vi "New_GraphDispWithTime.vi"() -> ()   [LabVIEW 2016, in "PanelSplitForDisplay.lvclass"]
uses:
  PanelSplit/PanelSplitForDisplay.lvclass
  PanelSplit/PanelObject/PanelObject.lvclass
  <vilib>/Utility/error.llb/DialogType.ctl
  PanelSplit/PanelDataNode/PanelDataNode.lvclass
  Architecture/Queue Management/ARC_Queue Create_Single.vi
  Architecture/Queue Management/ARC_Queue Remove Element.vi
  Ctrls/GlobeVaribles.vi
  Architecture/Queue Management/ARC_Queue Insert Element.vi
  Architecture/Queue Management/ARC_Queue Destroy_Single.vi
panel:
  out "Y Scale.Scale Fit":u8
  out "size(s)":i32
  in  "Node*":refnum<data-value>
  out "Waveform Chart":waveform(dbl)(graph)
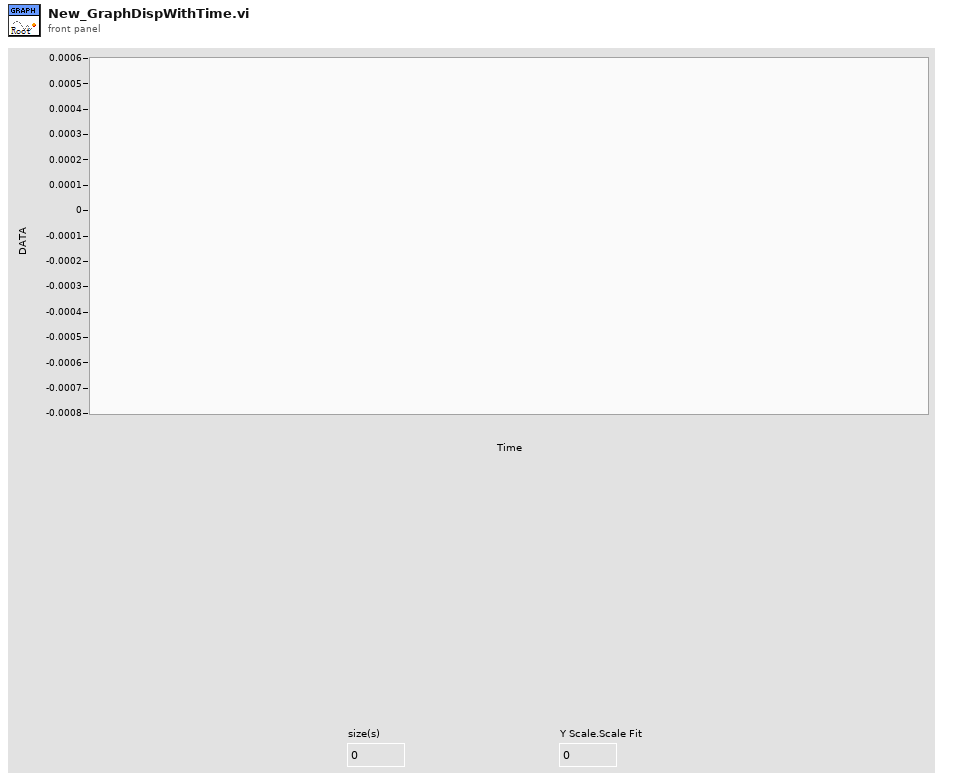
[diagram p1: front panel]
types:
  T1 = cluster{"error":errorcluster, "Event":string, "Data":variant, "Q_Local":string, "Graph":refnum<vi>, "Q_Caller":string}
  T2 = typedef "DialogType.ctl" = u16
  T3 = typedef "LVRectTypeDef.ctl" = cluster{"Left":i16, "Top":i16, "Right":i16, "Bottom":i16}
  T4 = typedef "PanelSplitForDisplay.lvclass/ViValueCtl.ctl" = cluster{"CHTag":string, "GraphProperts":cluster{"YMax":dbl, "YMin":dbl, "ScaleFit":u8}, "CHUnit":string, "CHName":string, "CHValue":string, "CHAlias":string}
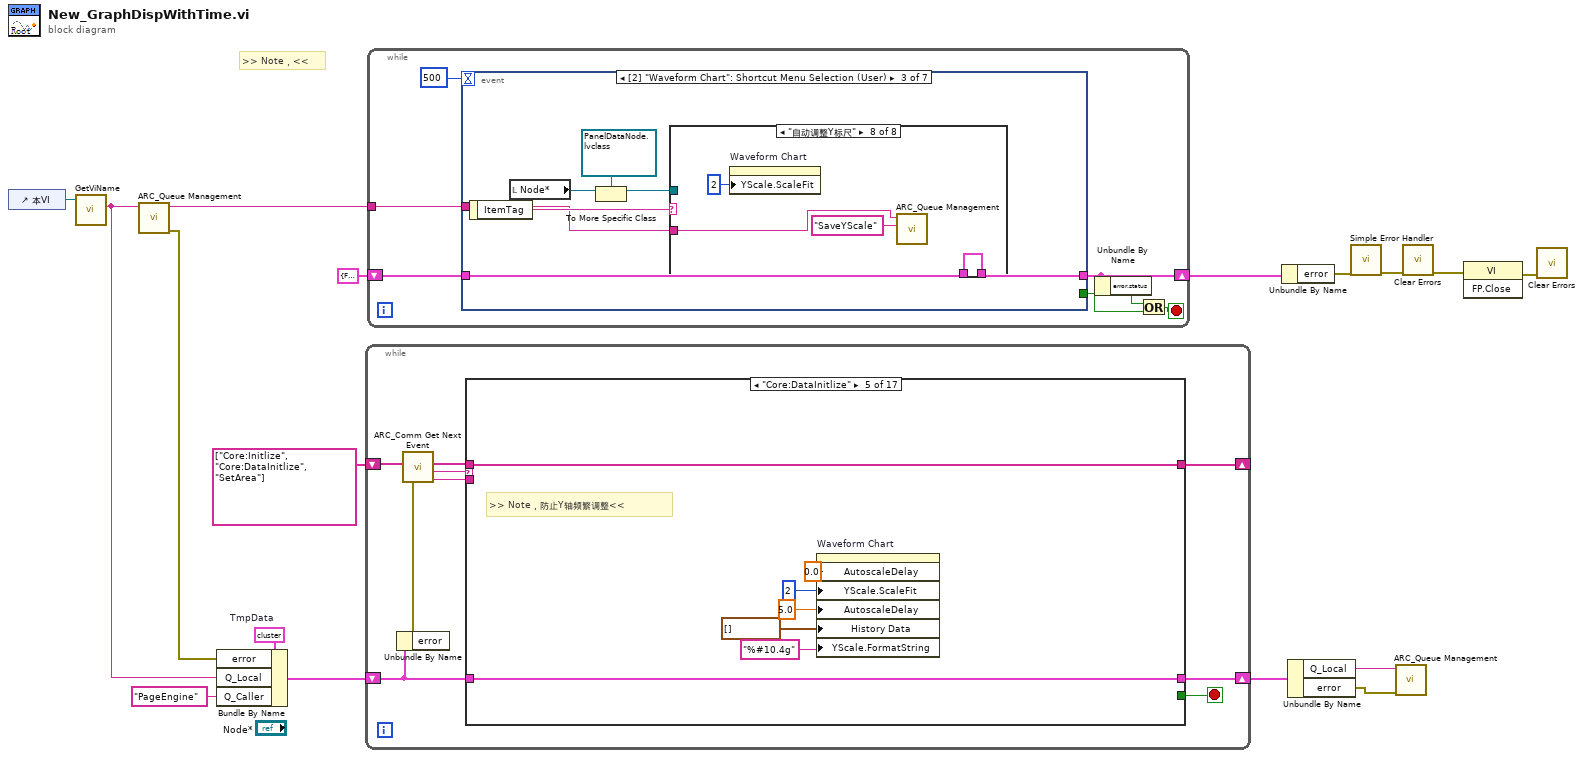
[diagram p0: block diagram]
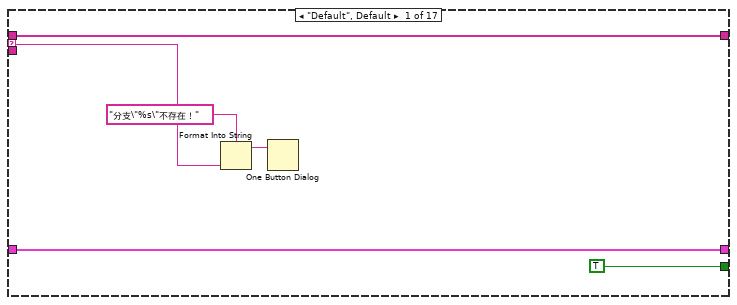
[diagram p2: hidden frame]
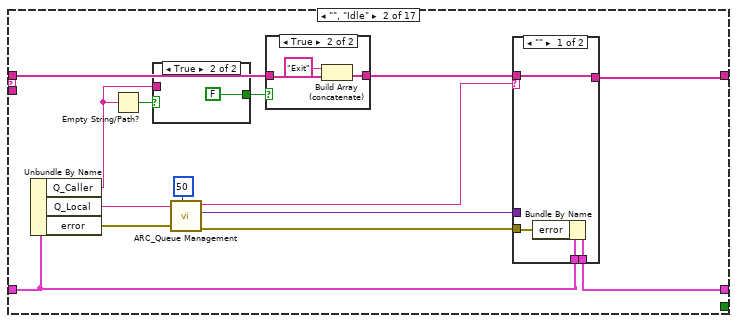
[diagram p3: hidden frame]
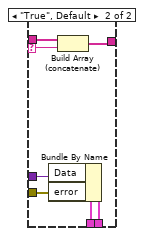
[diagram p4: hidden frame]
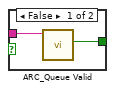
[diagram p6: hidden frame]
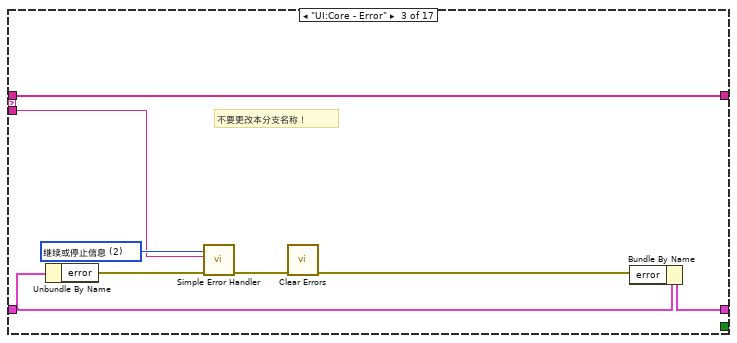
[diagram p7: hidden frame]
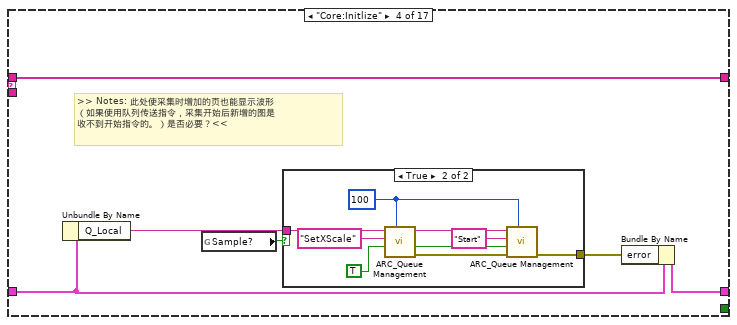
[diagram p8: hidden frame]
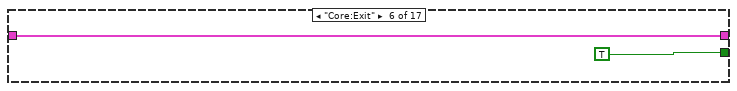
[diagram p10: hidden frame]
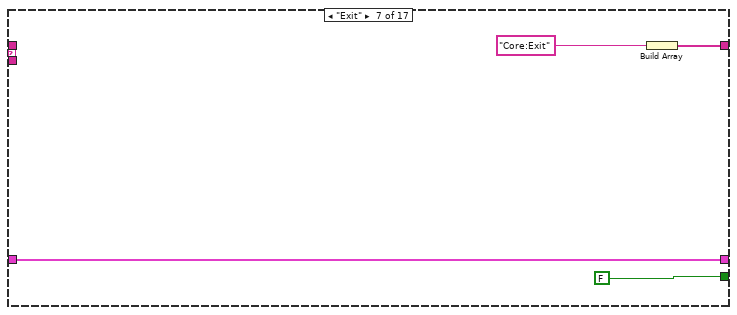
[diagram p11: hidden frame]
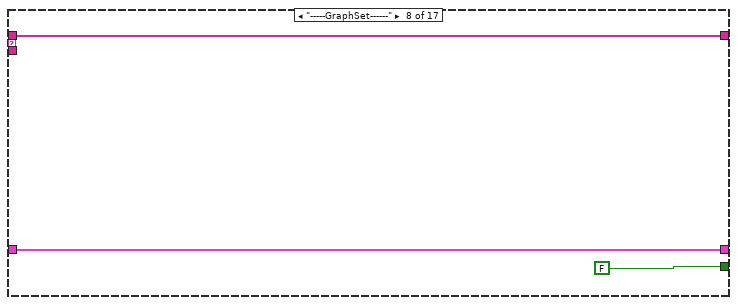
[diagram p12: hidden frame]
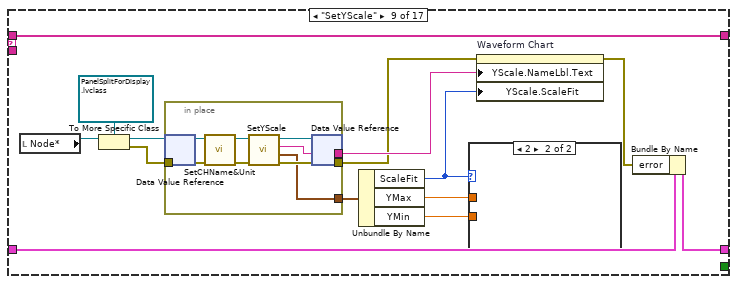
[diagram p13: hidden frame]
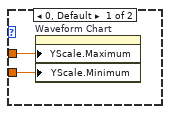
[diagram p14: hidden frame]
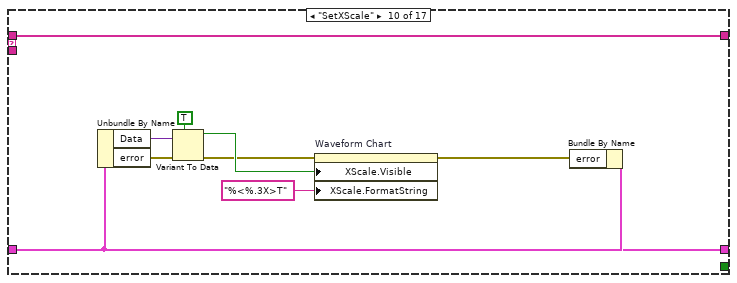
[diagram p15: hidden frame]
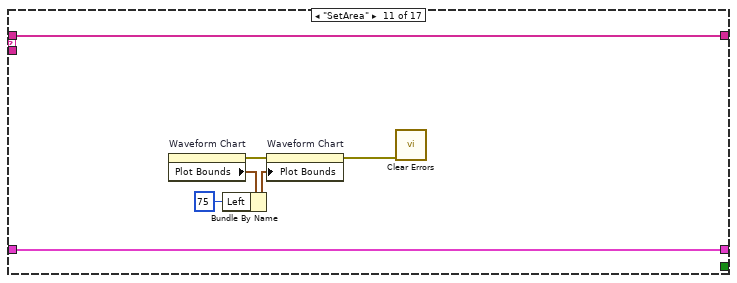
[diagram p16: hidden frame]
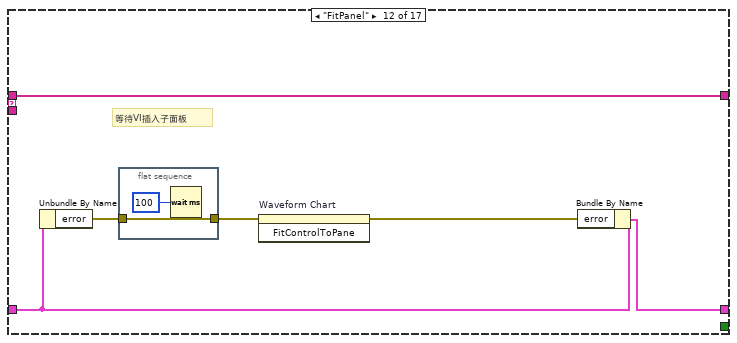
[diagram p17: hidden frame]
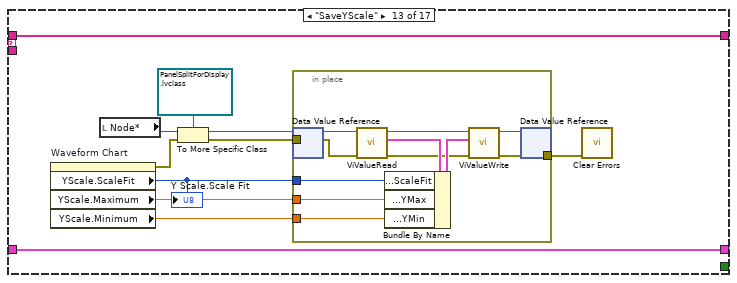
[diagram p18: hidden frame]
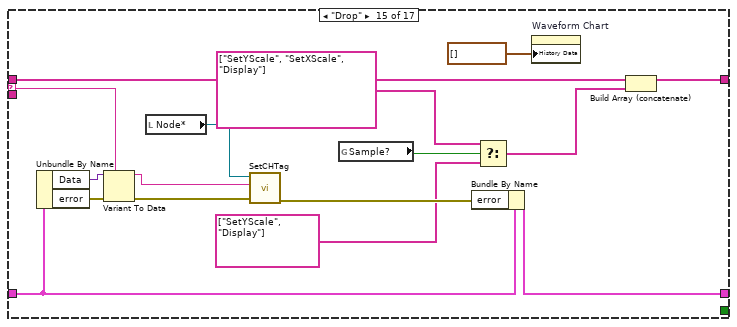
[diagram p20: hidden frame]
diagram:
  w14 = T1 {"error"={"status"=FALSE, "code"=0, "source"=""}, "Event"="", "Data"=variant, "Q_Local"="", "Graph"=refnum, "Q_Caller"=""}  # TmpData
  # ">> Note，<<"
  n1 = control-ref of="本VI"() -> (w7:refnum<vi>)
  n2 = call "GetViName.vi"("VI*"=w7) -> ("VI Name"=w10:string)  [unwired: 9 in, 1 out]
  n3 = call-poly "ARC_Queue Management.vi"("Queue Name"=w10) -> ("error out"=w11:errorcluster)  [unwired: 8 in, 2 out]
  n4 = Bundle By Name(cluster=w14, "error"=w11, "Q_Local"=w10, "Q_Caller"="PageEngine") -> (w13:T1)
  n5 = while {
    shift-right: [w21] -> w15
    shift-left: w13 -> [w22]
    shift-right: [w20] -> _
    shift-left: string[] ["Core:Initlize", "Core:DataInitlize", "SetArea"] ("event queue out") -> [w17]
    stop <- w24 stop-if-true
    n6 = Unbundle By Name(w22) -> ("error"=w23:errorcluster)
    n7 = call "ARC_Comm Get Next Event.vi"("error in (no error)"=w23, "event queue in"=w17) -> ("prev event"=w25:string, "next event"=w19:string, "event queue out"=w18:string[])  [unwired: 4 in]
    n8 = case shown="\"Core:DataInitlize\"" w19 {
      selector: w19 -> [w29 _ _ _ _ _ _ _ _ _ _ _ _ _ w175 _ _]
      tunnel: w18 -> [w30 w38 w71 w72 w91 _ _ w98 w114 w134 w141 w147 w160 w172 w188 w192 w206]
      tunnel: w25 -> [_ _ w64 _ _ _ _ _ _ _ _ _ _ _ _ _ _]
      tunnel: [TRUE _ _ _ _ TRUE FALSE FALSE _ _ _ _ _ _ _ _ _] -> w24
      tunnel: w22 -> [w31 w33 w67 w76 w90 w92 w96 w99 w107 w131 w136 w143 w151 w173 w185 w197 w207]
      tunnel: [w31 w32 w66 w77 w90 w92 w96 w99 w106 w130 w136 w145 w151 w173 w183 w197 w207] -> w21
      tunnel: [w30 w40 w71 w72 w91 _ w94 w98 w114 w134 w141 w147 w160 w172 w187 w191 w206] -> w20
      frame "Default", Default {
        n9 = Format Into String(format string="分支\"%s\"不存在！" ("格式字符串"), w29) -> (resulting string=w28:string)  [unwired: 2 in, 1 out]
        n10 = One Button Dialog(message=w28) -> ()  [unwired: 1 in, 1 out]
      }
      frame "", "Idle" {
        n11 = Unbundle By Name(w33) -> ("Q_Caller"=w43:string, "Q_Local"=w45:string, "error"=w42:errorcluster)
        n12 = Empty String/Path?(string/path=w43) -> (empty?=w44:bool)
        n13 = case shown="True" w44 {
          tunnel: [w61 FALSE ("Not Exist?")] -> w39
          tunnel: w43 -> [w62 _]
          frame False {
            n14 = call "ARC_Queue Valid.vi"("Queue Name(unamed)"=w62) -> ("Not Exist?"=w61:bool)  [unwired: 8 in, 2 out]
          }
          frame True {
          }
        }
        n15 = call-poly "ARC_Queue Management.vi"("Time out(-1)_queue out"=50 ("Time out(-1)"), "error in (no error)"=w42, "Queue Name(unamed)"=w45) -> ("error out"=w34:errorcluster, "Data"=w35:variant, "Event"=w36:string)  [unwired: 5 in, 1 out]
        n16 = case shown="True" w39 {
          tunnel: w38 -> [w57 w60]
          tunnel: [w57 w58] -> w37
          frame False {
          }
          frame True {
            n17 = Build Array (concatenate)("Exit" ("Event"), w60) -> (w58:string[])
          }
        }
        n18 = case shown="\"\"" w36 {
          selector: w36 -> [_ w54]
          tunnel: [w49 w56] -> w40
          tunnel: w37 -> [w49 w55]
          tunnel: w35 -> [_ w53]
          tunnel: w34 -> [w46 w52]
          tunnel: w33 -> [w48 w51]
          tunnel: [w47 w50] -> w32
          frame "" {
            n19 = Bundle By Name(cluster=w48, "error"=w46) -> (w47:T1)
          }
          frame "True", Default {
            n20 = Bundle By Name(cluster=w51, "Data"=w53, "error"=w52) -> (w50:T1)
            n21 = Build Array (concatenate)(w55, w54) -> (w56:string[])
          }
        }
      }
      frame "UI:Core - Error" {
        w65 = T2 2 items=["无对话框", "确定信息", "继续或停止信息", "确定信息＋警告", "继续/停止+警告"] ("type of dialog (OK msg:1)")
        # "不要更改本分支名称！"
        n22 = Unbundle By Name(w67) -> ("error"=w68:errorcluster)
        n23 = call <vilib>:"Simple Error Handler.vi"("error source (\" \")"=w64, "type of dialog (OK msg:1)"=w65, "error in (no error)"=w68) -> ("error out"=w69:errorcluster)  [unwired: 2 in, 4 out]
        n24 = call <vilib>:"Clear Errors.vi"("error in (no error)"=w69) -> ("error out"=w70:errorcluster)  [unwired: 5 in, 1 out]
        n25 = Bundle By Name(cluster=w67, "error"=w70) -> (w66:T1)
      }
      frame "Core:Initlize" {
        # ">> Notes: 此处使采集时增加的页也能显示波形\n（如果使用队列传送指令，采集开始后新增的图是\n收不到开始指令的。）是否必要？<<"
        n26 = Unbundle By Name(w76) -> ("Q_Local"=w75:string)
        n27 = global read "GlobeVaribles.vi" "Sample?"() -> (w73:bool)
        n28 = case shown="True" w73 {
          tunnel: w75 -> [_ w79]
          tunnel: [_ w82] -> w74
          frame False {
          }
          frame True {
            w81 = 100 ("Time out(-1)_queue in")
            w78 = TRUE
            n29 = call-poly "ARC_Queue Management.vi"("Time out(-1)_queue in"=w81, "Data"=w78, "Event"="SetXScale", "Queue Name(unamed)"=w79) -> ("error out"=w83:errorcluster)  [unwired: 6 in, 1 out]
            n30 = call-poly "ARC_Queue Management.vi"("Time out(-1)_queue in"=w81, "error in (no error)"=w83, "Data"=w78, "Event"="Start", "Queue Name(unamed)"=w79) -> ("error out"=w82:errorcluster)  [unwired: 5 in, 1 out]
          }
        }
        n31 = Bundle By Name(cluster=w76, "error"=w74) -> (w77:T1)
      }
      frame "Core:DataInitlize" {
        # ">> Note，防止Y轴频繁调整<<"
        n32 = property on="Waveform Chart" class="WFChart (strict)"("AutoscaleDelay"=sgl 0.0 ("自动调整标尺延迟"), "YScale.ScaleFit"=u8 2 ("Y标尺.标尺调节"), "AutoscaleDelay"=sgl 5.0 ("自动调整标尺延迟"), "History Data"=waveform(dbl)[] [] ("历史数据"), "YScale.FormatString"="%#10.4g" ("Y标尺.格式字符串")) -> ()  [unwired: 2 in, 2 out]
      }
      frame "Core:Exit" {
      }
      frame "Exit" {
        n33 = Build Array("Core:Exit" ("Remaining States")) -> (w94:string[])
      }
      frame "-----GraphSet------" {
      }
      frame "SetYScale" {
        n34 = local read "Node*"() -> (w113:refnum<data-value>)
        n35 = To More Specific Class(target class=refnum<data-value> refnum ("数据值引用"), reference=w113) -> (specific class reference=w112:refnum<data-value>, error out=w110:errorcluster)  [unwired: 1 in]
        n36 = in-place {
          in-place-border: w110 -> [w119]
          in-place-border: [w123] -> w109
          in-place-border: [w122] -> w108
          in-place-border: [w117] -> w105
          n37 = in-place-dvr #1(w112) -> (w121:refnum<class "PanelSplitForDisplay.lvclass">)  [unwired: 1 out]
          n38 = call "SetCHName&Unit.vi"("error in (no error)"=w119, "PanelSplitForDisplay 输入"=w121) -> ("error out"=w118:errorcluster, "PanelSplitForDisplay 输出"=w120:refnum<class "PanelSplitForDisplay.lvclass">)  [unwired: 8 in]
          n39 = call "SetYScale.vi"("error in"=w118, "PanelSplitForDisplay 输入"=w120) -> ("error out"=w122:errorcluster, "GraphProperts"=w117:cluster{"YMax":dbl, "YMin":dbl, "ScaleFit":u8}, "YLable"=w123:string, "PanelSplitForDisplay 输出"=w124:refnum<class "PanelSplitForDisplay.lvclass">)  [unwired: 6 in]
          n40 = in-place-dvr #1(w124) -> ()  [unwired: 2 out]
        }
        n41 = Unbundle By Name(w105) -> ("ScaleFit"=w104:u8, "YMax"=w103:dbl, "YMin"=w102:dbl)
        n42 = case shown="2" w104 {
          tunnel: w103 -> [w116 _]
          tunnel: w102 -> [w115 _]
          frame 0, Default {
            n43 = property on="Waveform Chart" class="WFChart (strict)"("YScale.Maximum"=w116, "YScale.Minimum"=w115) -> ()  [unwired: 2 in, 2 out]
          }
          frame 2 {
          }
        }
        n44 = property on="Waveform Chart" class="WFChart (strict)"(error in=w108, "YScale.NameLbl.Text"=w109, "YScale.ScaleFit"=w104) -> (error out=w101:errorcluster)  [unwired: 1 in, 1 out]
        n45 = Bundle By Name(cluster=w107, "error"=w101) -> (w106:T1)
      }
      frame "SetXScale" {
        n46 = Unbundle By Name(w131) -> ("Data"=w132:variant, "error"=w126:errorcluster)
        n47 = Variant To Data(error in=w126, type=TRUE ("X标尺.可见"), Variant=w132) -> (data=w129:bool, error out=w128:errorcluster)
        n48 = property on="Waveform Chart" class="WFChart (strict)"(error in=w128, "XScale.Visible"=w129, "XScale.FormatString"="%<%.3X>T" ("X Scale.Format String")) -> (error out=w127:errorcluster)  [unwired: 1 in, 1 out]
        n49 = Bundle By Name(cluster=w131, "error"=w127) -> (w130:T1)
      }
      frame "SetArea" {
        n50 = property on="Waveform Chart" class="WFChart (strict)"() -> (error out=w137:errorcluster, "Plot Bounds"=w140:T3)  [unwired: 2 in, 1 out]
        n51 = Bundle By Name(cluster=w140, "Left"=i16 75 ("left")) -> (w139:T3)
        n52 = property on="Waveform Chart" class="WFChart (strict)"(error in=w137, "Plot Bounds"=w139) -> (error out=w135:errorcluster)  [unwired: 1 in, 1 out]
        n53 = call <vilib>:"Clear Errors.vi"("error in (no error)"=w135) -> ()  [unwired: 5 in, 2 out]
      }
      frame "FitPanel" {
        # "等待VI插入子面板"
        n54 = Unbundle By Name(w143) -> ("error"=w142:errorcluster)
        n55 = flat-sequence {
          tunnel: [w148] -> w144
          tunnel: w142 -> [w148]
          frame #0 {
            n56 = Wait (ms)(milliseconds to wait=u32 100 ("等待时间（毫秒）")) -> ()  [unwired: 1 out]
          }
        }
        n57 = invoke on="Waveform Chart" class="WFChart (严格)" method="FitControlToPane"(error in=w144) -> (error out=w146:errorcluster)  [unwired: 2 in, 2 out]
        n58 = Bundle By Name(cluster=w143, "error"=w146) -> (w145:T1)
      }
      frame "SaveYScale" {
        n59 = property on="Waveform Chart" class="WFChart (strict)"() -> (error out=w152:errorcluster, "YScale.ScaleFit"=w155:u8, "YScale.Maximum"=w154:dbl, "YScale.Minimum"=w153:dbl)  [unwired: 2 in, 1 out]
        "Y Scale.Scale Fit" <- w155
        n60 = local read "Node*"() -> (w159:refnum<data-value>)
        n61 = To More Specific Class(target class=refnum<data-value> refnum ("数据值引用"), reference=w159, error in=w152) -> (specific class reference=w156:refnum<data-value>, error out=w157:errorcluster)
        n62 = in-place {
          in-place-border: w157 -> [w163]
          in-place-border: w155 -> [w166]
          in-place-border: w154 -> [w165]
          in-place-border: w153 -> [w164]
          in-place-border: [w161] -> _
          n63 = in-place-dvr #2(w156) -> (w171:refnum<class "PanelSplitForDisplay.lvclass">)  [unwired: 1 out]
          n64 = call "ViValueRead.vi"("error in (no error)"=w163, "PanelSplitForDisplay 输入"=w171) -> ("error out"=w162:errorcluster, "ViValue"=w168:T4, "PanelSplitForDisplay 输出"=w170:refnum<class "PanelSplitForDisplay.lvclass">)  [unwired: 7 in]
          n65 = Bundle By Name(cluster=w168, "GraphProperts.ScaleFit"=w166, "GraphProperts.YMax"=w165, "GraphProperts.YMin"=w164) -> (w167:T4)
          n66 = call "ViValueWrite.vi"("error in (no error)"=w162, "ViValue"=w167, "PanelSplitForDisplay 输入"=w170) -> ("error out"=w161:errorcluster, "PanelSplitForDisplay 输出"=w169:refnum<class "PanelSplitForDisplay.lvclass">)  [unwired: 7 in]
          n67 = in-place-dvr #2(w169) -> (w150:errorcluster)  [unwired: 1 out]
        }
        n68 = call <vilib>:"Clear Errors.vi"("error in (no error)"=w150) -> ()  [unwired: 5 in, 2 out]
      }
      frame "----------------------" {
      }
      frame "Drop" {
        n69 = Unbundle By Name(w185) -> ("Data"=w176:variant, "error"=w184:errorcluster)
        n70 = Variant To Data(error in=w184, type=w175, Variant=w176) -> (data=w174:string, error out=w177:errorcluster)
        n71 = local read "Node*"() -> (w186:refnum<data-value>)
        n72 = call "SetCHTag.vi"("error in (no error)"=w177, "ChannelTag"=w174, "Node*"=w186) -> ("error out"=w182:errorcluster)  [unwired: 8 in]
        n73 = global read "GlobeVaribles.vi" "Sample?"() -> (w181:bool)
        n74 = Bundle By Name(cluster=w185, "error"=w182) -> (w183:T1)
        n75 = Select(t=string[] ["SetYScale", "SetXScale", "Display"] ("event queue out"), s=w181, f=string[] ["SetYScale", "Display"] ("event queue out")) -> (s? t:f=w178:string[])
        n76 = property on="Waveform Chart" class="WFChart (strict)"("History Data"=waveform(dbl)[] [] ("历史数据")) -> ()  [unwired: 2 in, 2 out]
        n77 = Build Array (concatenate)(w188, w178) -> (w187:string[])
      }
      frame "Display" {
        # ">> Note，读取数据的循环速度应为写入速度的两倍以上，程序中已做了防重复读取处理\n需测试是否可行<<"
        n78 = local read "Node*"() -> (w196:refnum<data-value>)
        n79 = To More Specific Class(target class=refnum<data-value> refnum ("数据值引用"), reference=w196) -> (specific class reference=w195:refnum<data-value>, error out=w193:errorcluster)  [unwired: 1 in]
        n80 = case shown="No Error" w193 {
          tunnel: w195 -> [w198 _]
          frame No Error {
            n81 = in-place {
              n82 = in-place-dvr #3(w198) -> (w204:refnum<class "PanelSplitForDisplay.lvclass">, w201:errorcluster)
              n83 = call "GetSampleData.vi"("error in"=w201, "PanelSplitForDisplay.lvclass"=w204) -> ("Display?"=w200:bool, "signal out"=w202:waveform(dbl), "PanelSplitForDisplay.lvclass 2"=w203:refnum<class "PanelSplitForDisplay.lvclass">, "size(s)"=→"size(s)":i32)  [unwired: 3 in, 1 out]
              n84 = case shown="True" w200 {
                tunnel: w202 -> [_ w205]
                frame False {
                }
                frame True {
                  "Waveform Chart" <- w205
                }
              }
              n85 = in-place-dvr #3(w203) -> ()  [unwired: 2 out]
            }
          }
          frame Error {
          }
        }
        n86 = Build Array (concatenate)(w192, string[] ["Idle", "Display", "SetArea"] ("array")) -> (w191:string[])
      }
      frame "Stop" {
      }
    }
  }
  n87 = while {
    tunnel: w10 -> [w214]
    shift-right: [w209] -> w8
    shift-left: cluster{"Float?":bool, "error":errorcluster} {"Float?"=FALSE, "error"={"status"=FALSE, "code"=0, "source"=""}} -> [w213]
    stop <- w211 stop-if-true
    n88 = event shown="[2] \"Waveform Chart\": Shortcut Menu Selection (User)" {
      selector: _ -> [_ _ _ _ _ _ _]
      dyn-events: _ -> [_ _ _ _ _ _ _]
      timeout: 500 -> [_ _ _ _ _ _ _]
      tunnel: [w215 _ _ _ _ _ FALSE] -> w212
      tunnel: w214 -> [w218 _ w228 w266 _ w270 _]
      tunnel: w213 -> [w216 w221 w230 w267 w268 w277 w281]
      tunnel: [w216 w221 w229 w267 w268 w272 w280] -> w209
      event Timeout {
        n89 = event-data() -> ()  [unwired: 1 in, 2 out]
        n90 = Unbundle By Name(w216) -> ("error"=w217:errorcluster)
        n91 = call-poly "ARC_Queue Management.vi"("error in"=w217, "Queue Name"=w218) -> ("Created New?"=w215:bool)  [unwired: 7 in, 2 out]
      }
      event "Waveform Chart": Shortcut Menu Activation? {
        n92 = event-data() -> ("MenuRef"=w225:refnum<k9>)  [unwired: 1 in]
        n93 = Unbundle By Name(w221) -> ("Float?"=w220:bool)
        n94 = Not(x=w220) -> (.not. x?=w219:bool)
        n95 = Select(t=string[] ["浮动", "自动调整Y标尺"] ("项名称"), s=w219, f=string[] ["返回"]) -> (s? t:f=w223:string[])
        n96 = Delete Menu Items(9:w225) -> (0:w226:errorcluster, 3:w227:refnum<k9>)  [unwired: 3 in]
        n97 = Insert Menu Items(6:w226, 7:w223, 8:w223, 9:w227) -> ()  [unwired: 2 in, 3 out]
        n98 = event-data() -> ()  [unwired: 2 in, 1 out]
      }
      event "Waveform Chart": Shortcut Menu Selection (User) {
        n99 = event-data() -> ("ItemTag"=w232:string)  [unwired: 1 in]
        n100 = local read "Node*"() -> (w233:refnum<data-value>)
        n101 = To More Specific Class(target class=refnum<data-value> refnum ("Node*"), reference=w233) -> (specific class reference=w231:refnum<data-value>)  [unwired: 1 in, 1 out]
        n102 = case shown="\"自动调整Y标尺\"" w232 {
          tunnel: w231 -> [_ w237 w241 w248 _ _ _ _]
          tunnel: w230 -> [w235 w236 w240 w247 w253 w255 w256 w260]
          tunnel: [w235 w236 w239 w245 w253 w255 w256 w260] -> w229
          tunnel: w228 -> [_ _ _ _ _ _ _ w257]
          frame "假", Default {
          }
          frame "删除" {
            n103 = call "Q_Delete.vi"("ChildNode*"=w237) -> ()  [unwired: 10 in, 1 out]
          }
          frame "浮动" {
            n104 = in-place {
              n105 = in-place-dvr #4(w241) -> (w244:refnum<class "PanelDataNode.lvclass">, w242:errorcluster)
              n106 = call "RefreshPanel.vi"("error in (no error)"=w242, "PanelDataNode 输入"=w244) -> ("PanelDataNode 输出"=w243:refnum<class "PanelDataNode.lvclass">)  [unwired: 8 in, 1 out]
              n107 = in-place-dvr #4(w243) -> ()  [unwired: 2 out]
            }
            n108 = Bundle By Name(cluster=w240, "Float?"=TRUE) -> (w239:cluster{"Float?":bool, "error":errorcluster})
          }
          frame "返回" {
            n109 = in-place {
              n110 = in-place-dvr #5(w248) -> (w251:refnum<class "PanelDataNode.lvclass">, w249:errorcluster)
              n111 = call "BackToPanel.vi"("error in (no error)"=w249, "PanelDataNode 输入"=w251) -> ("PanelDataNode 输出"=w250:refnum<class "PanelDataNode.lvclass">)  [unwired: 8 in, 1 out]
              n112 = in-place-dvr #5(w250) -> ()  [unwired: 2 out]
            }
            n113 = Bundle By Name(cluster=w247, "Float?"=FALSE) -> (w245:cluster{"Float?":bool, "error":errorcluster})
          }
          frame "显示" {
            n114 = property on="Waveform Chart" class="WFChart (strict)"("XScale.Visible"=TRUE ("X标尺.可见")) -> ()  [unwired: 2 in, 2 out]
          }
          frame "隐藏" {
            n115 = property on="Waveform Chart" class="WFChart (strict)"("XScale.Visible"=FALSE ("X标尺.可见")) -> ()  [unwired: 2 in, 2 out]
          }
          frame "Fit" {
            n116 = invoke on="Waveform Chart" class="WFChart (严格)" method="FitControlToPane"() -> ()  [unwired: 3 in, 3 out]
          }
          frame "自动调整Y标尺" {
            n117 = property on="Waveform Chart" class="WFChart (strict)"("YScale.ScaleFit"=u8 2 ("Y标尺.标尺调节")) -> ()  [unwired: 2 in, 2 out]
            n118 = call-poly "ARC_Queue Management.vi"("Event"="SaveYScale", "Queue Name(unamed)"=w257) -> ()  [unwired: 8 in, 2 out]
          }
        }
      }
      event "Waveform Chart": Drop {
        w262 = "ChannelInfo" ("数据名称")
        n119 = event-data() -> ()  [unwired: 1 in, 1 out]
        n120 = Get Drag Drop Data(8:w262, 9:w262) -> (3:w261:string)  [unwired: 1 in, 1 out]
        n121 = call-poly "ARC_Queue Management.vi"("Time out(-1)_queue in"=50, "Data"=w261, "Event"="Drop", "Queue Name(unamed)"=w266) -> ()  [unwired: 6 in, 2 out]
        n122 = event-data("Accepted?"=TRUE ("接受？")) -> ()  [unwired: 1 in, 1 out]
      }
      event "Waveform Chart": Drag Enter {
        n123 = event-data() -> ()  [unwired: 1 in, 1 out]
        n124 = event-data("Accepted?"=TRUE ("接受？")) -> ()  [unwired: 1 in, 1 out]
      }
      event "Waveform Chart": Scale Range Change {
        n125 = event-data() -> ()  [unwired: 1 in, 2 out]
        n126 = Unbundle By Name(w277) -> ("error"=w276:errorcluster)
        n127 = property on="Waveform Chart" class="WFChart (strict)"("YScale.ScaleFit"=u8 0 ("Y标尺.标尺调节")) -> ()  [unwired: 2 in, 2 out]
        n128 = call-poly "ARC_Queue Management.vi"("error in (no error)"=w276, "Event"="SetArea", "Queue Name(unamed)"=w270) -> ("error out"=w274:errorcluster)  [unwired: 7 in, 1 out]
        n129 = call-poly "ARC_Queue Management.vi"("error in (no error)"=w274, "Event"="SaveYScale", "Queue Name(unamed)"=w270) -> ("error out"=w271:errorcluster)  [unwired: 7 in, 1 out]
        n130 = Bundle By Name(cluster=w277, "error"=w271) -> (w272:cluster{"Float?":bool, "error":errorcluster})
      }
      event Panel Close? {
        n131 = event-data() -> ()  [unwired: 1 in, 1 out]
        n132 = local read "Node*"() -> (w282:refnum<data-value>)
        n133 = To More Specific Class(target class=refnum<data-value> refnum ("Node*"), reference=w282) -> (specific class reference=w284:refnum<data-value>, error out=w283:errorcluster)  [unwired: 1 in]
        n134 = case shown="No Error" w283 {
          selector: w283 -> [w289 w295]
          tunnel: w284 -> [w290 _]
          tunnel: [w288 w295] -> _
          frame No Error {
            n135 = in-place {
              in-place-border: w289 -> [w292]
              in-place-border: [w291] -> w288
              n136 = in-place-dvr #6(w290) -> (w294:refnum<class "PanelDataNode.lvclass">)  [unwired: 1 out]
              n137 = call "BackToPanel.vi"("error in (no error)"=w292, "PanelDataNode 输入"=w294) -> ("error out"=w291:errorcluster, "PanelDataNode 输出"=w293:refnum<class "PanelDataNode.lvclass">)  [unwired: 8 in]
              n138 = in-place-dvr #6(w293) -> ()  [unwired: 2 out]
            }
          }
          frame Error {
          }
        }
        n139 = Bundle By Name(cluster=w281, "Float?"=FALSE) -> (w280:cluster{"Float?":bool, "error":errorcluster})
        n140 = event-data("Discard?"=TRUE ("放弃？")) -> ()  [unwired: 1 in, 1 out]
      }
    }
    n141 = Unbundle By Name(w209) -> ("error.status"=w208:bool)
    n142 = Or(x=w208, y=w212) -> (x .or. y?=w211:bool)
  }
  n143 = Unbundle By Name(w8) -> ("error"=w5:errorcluster)
  n144 = Unbundle By Name(w15) -> ("Q_Local"=w12:string, "error"=w16:errorcluster)
  n145 = call <vilib>:"Simple Error Handler.vi"("error in (no error)"=w5) -> ("error out"=w3:errorcluster)  [unwired: 4 in, 4 out]
  n146 = call-poly "ARC_Queue Management.vi"("error in (no error)"=w16, "Queue Name(unamed)"=w12) -> ()  [unwired: 7 in, 3 out]
  n147 = call <vilib>:"Clear Errors.vi"("error in (no error)"=w3) -> ("error out"=w2:errorcluster)  [unwired: 5 in, 1 out]
  n148 = invoke class="VI" method="FP.Close"(error in=w2) -> (error out=w4:errorcluster)  [unwired: 2 in, 2 out]
  n149 = call <vilib>:"Clear Errors.vi"("error in (no error)"=w4) -> ()  [unwired: 5 in, 2 out]
